vi "Start Group.vi"(8 "error in (no error)":errorcluster {"code" format="Error %.0f"}, 10 "Group":string, 11 "VIDoc Printer - Confluence In":refnum<class "VIDoc Printer - Confluence.lvclass">) -> (0 "error out":errorcluster {"code" format="Error %.0f"}, 3 "VIDoc Printer - Confluence Out":refnum<class "VIDoc Printer - Confluence.lvclass">)   [LabVIEW 2023, in "VIDoc Printer - Confluence.lvlib" / "VIDoc Printer - Confluence.lvclass"]
uses:
  VIDoc Printer - Confluence.lvclass
  Printer/VIDoc Printer.lvclass
  VIDoc Printer - Confluence.lvclass/VIDoc Printer - Confluence.ctl
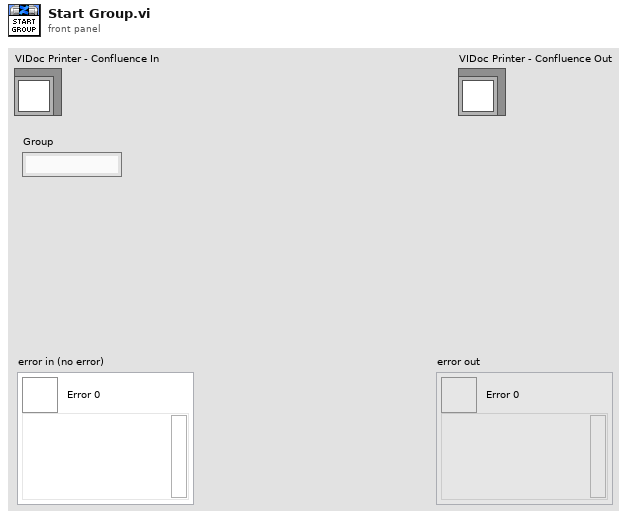
[diagram p1: front panel]
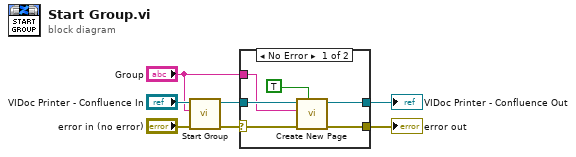
[diagram p0: block diagram]
diagram:
  n1 = call-parent "Start Group.vi"("error in (no error)"="error in (no error)", "Group"="Group", "VIDoc Printer In"="VIDoc Printer - Confluence In") -> ("error out"=w5:errorcluster, "VIDoc Printer Out"=w4:refnum<class "VIDoc Printer - Confluence.lvclass">)  [unwired: 7 in]
  n2 = case shown="No Error" w5 {
    selector: w5 -> [w12 w15]
    tunnel: [w11 w15] -> w1
    tunnel: [w10 w14] -> w2
    tunnel: w4 -> [w13 w14]
    tunnel: "Group" -> [w9 _]
    frame No Error {
      n3 = call "Create New Page.vi"("Update Current Page (F)"=TRUE, "error in (no error)"=w12, "Name"=w9, "VIDoc Printer - Confluence In"=w13) -> ("error out"=w11:errorcluster, "VIDoc Printer - Confluence Out"=w10:refnum<class "VIDoc Printer - Confluence.lvclass">)  [unwired: 4 in, 2 out]
    }
    frame Error {
    }
  }
  "error out" <- w1
  "VIDoc Printer - Confluence Out" <- w2
